vi "StatusRecord.vi"(8 "error in (no error)":errorcluster, 10 "Event Info":T1, 11 "new file path (Not A Path if cancelled) in":path) -> (0 "error out":errorcluster, 3 "new file path (Not A Path if cancelled) out":path)   [LabVIEW 2016]
uses:
  <vilib>/Utility/file.llb/Write Delimited Spreadsheet (string).vi
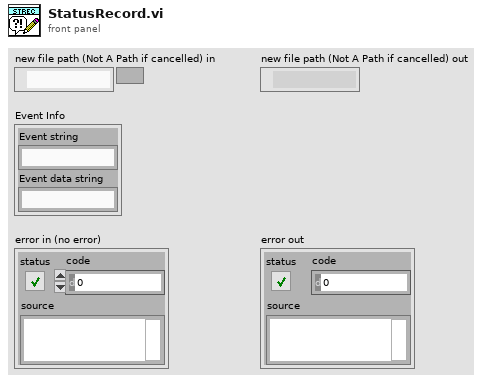
[diagram p1: front panel]
types:
  T1 = cluster{"Event string":string, "Event data string":string}
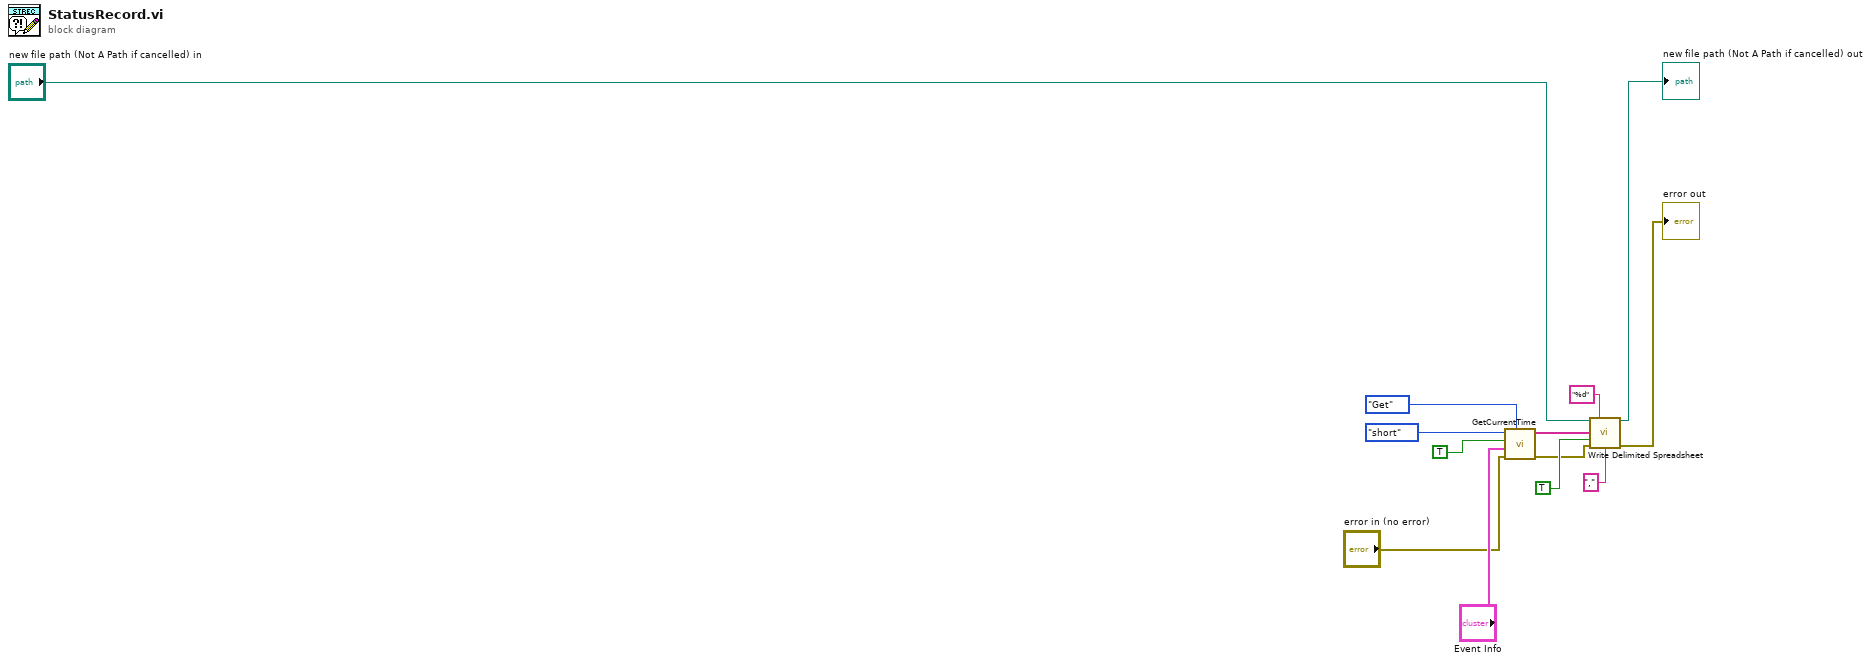
[diagram p0: block diagram]
diagram:
  n1 = call "GetCurrentTime.vi"("Date Operation (Get)"=enum16{"Get", "None (Future)"}."Get" ("Enum"), "error constant"="error in (no error)", "Event Information"="Event Info", "want seconds? (F)"=TRUE, "date format (0)"=enum16{"short", "long", "abbreviated"}."short") -> ("error IO"=w6:errorcluster, "Array"=w5:string[])  [unwired: 2 in, 1 out]
  n2 = call-poly <vilib>:"Write Delimited Spreadsheet.vi"("file path (dialog if empty)"="new file path (Not A Path if cancelled) in", "format (%s)"="%d" ("format string"), "1D data"=w5, "append to file? (new file:F)"=TRUE, "error in (no error)"=w6, "delimiter (\\t)"="," ("delimiter (\\t)")) -> ("new file path (Not A Path if cancelled)"=→"new file path (Not A Path if cancelled) out":path, "error out"=→"error out":errorcluster)  [unwired: 8 in]
